vi "Get image date.vi"(8 "error in (no error)":errorcluster, 11 "CCDCamera in":refnum<class "CCDCamera.lvclass">) -> (0 "error out":errorcluster, 3 "CCDCamera out":refnum<class "CCDCamera.lvclass">)   [LabVIEW 2018, in "CCDCamera.lvclass"]
uses:
  CCDCamera.lvclass
  C:/Users/observer/Desktop/SPARC4_ACS/SPARC4_ACS/Simulated_CCD_Camera/Simulated_CCD_Camera.lvclass
  Simulated_CCD_Camera/Simulated_CCD_Camera.lvclass
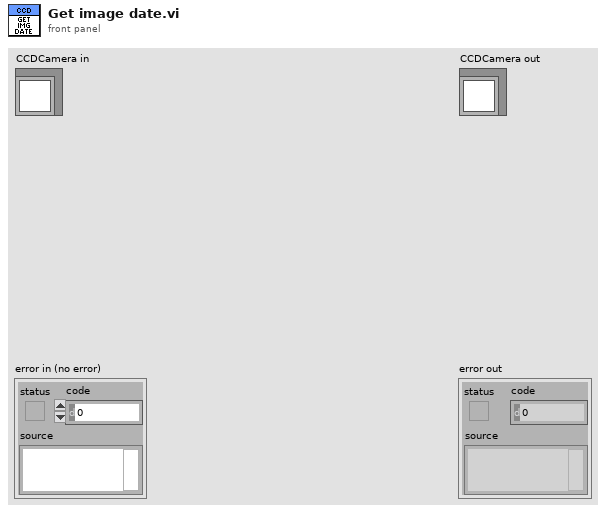
[diagram p1: front panel]
types:
  T1 = cluster{"CUBE_EXPOSURE_TIME":sgl, "CUBES_DONE":u16, "LAST_IMAGE_NAME":string, "DISK_SPACE":u16, "FRAMES_DONE":u16, "CCD_STATUS":string, "CURRENT_TEMPERATURE":i16, "TEMPERATURE_STATUS":string, "FRAME_EXPOSURE_TIME":dbl, "CCD_POWER_STATUS":bool, "SERIAL_NUMBER":u16, "ACQUIRING":bool}
  T2 = typedef "SYSTEMTIME structure typedef.ctl" = cluster{"Year":u16, "Month":u16, "DayOfWeek":u16, "Date":u16, "Hour":u16, "Minute":u16, "Second":u16, "Milliseconds":u16}
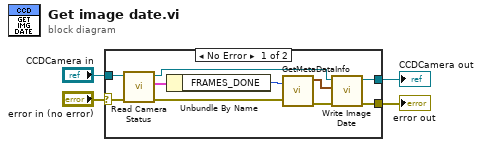
[diagram p0: block diagram]
diagram:
  n1 = case shown="No Error" "error in (no error)" {
    selector: "error in (no error)" -> [w9 w15]
    tunnel: [w13 w15] -> w3
    tunnel: "CCDCamera in" -> [w10 w16]
    tunnel: [w12 w16] -> w1
    frame No Error {
      n2 = call "Read Camera Status.vi"("error in (no error)"=w9, "CCDCamera in"=w10) -> ("error out"=w6:errorcluster, "Camera Status"=w8:T1, "CCDCamera out"=w5:refnum<class "CCDCamera.lvclass">)  [unwired: 7 in]
      n3 = Unbundle By Name(w8) -> ("FRAMES_DONE"=w7:u16)
      n4 = call <userlib>:"GetMetaDataInfo.vi"("index"=w7, "error in (no error)"=w6) -> ("SYSTEMTIME"=w11:T2, "error out"=w14:errorcluster)  [unwired: 2 out]
      n5 = call-dynamic "Write Image Date.vi"("error in (no error)"=w14, "SYSTEMTIME"=w11, "Simulated_CCD_Camera in"=w5) -> ("error out"=w13:errorcluster, "Simulated_CCD_Camera out"=w12:refnum<class "CCDCamera.lvclass">)  [unwired: 7 in]
    }
    frame Error {
    }
  }
  "error out" <- w3
  "CCDCamera out" <- w1
